vi "Event-Camera-amount.vi"(7 "# cameras":i32, 8 "error in (no error)":errorcluster, 10 "Data ref. in":refnum<data-value>, 11 "UI ref. in":refnum<data-value>) -> (0 "error out":errorcluster, 2 "Data ref.":refnum<data-value>, 3 "UI ref.":refnum<data-value>)   [LabVIEW 2013, in "CameraVision.lvlib" / "CV-UI.lvclass"]
uses:
  CV-UI.lvclass
  Main/CV-Main.lvclass
  Control-names.ctl
  Camera-selector.ctl
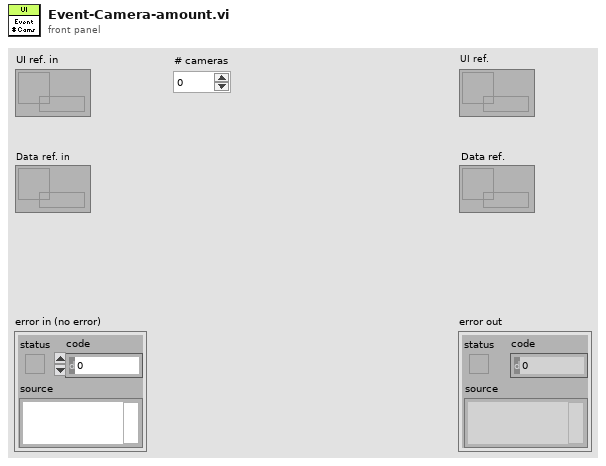
[diagram p1: front panel]
types:
  T1 = typedef "CameraVision.lvlib/CV-UI.lvclass/Control-names.ctl" = enum16{"Start acquisition", "Activate", "Stop acquisition", "Settings type", "Load settings", "Save settings", "Import images", "Camera selector", "Image type selector", "Batch browser", "Image refresh", "Parameter tabs", "Displays", "Processing tabs", "Processing selector", "Map characteristic", "Show info", "Manual trigger"}
  T2 = typedef "CameraVision.lvlib/CV-UI.lvclass/Camera-selector.ctl" = enum16{"Camera 1", "Camera 2"}
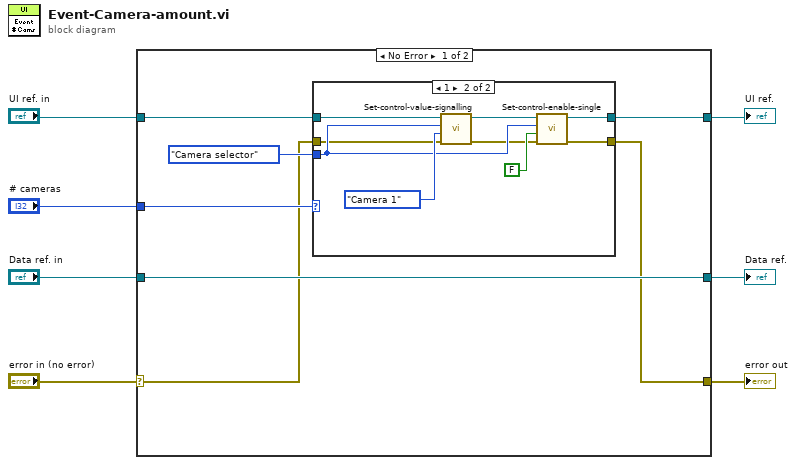
[diagram p0: block diagram]
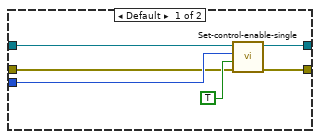
[diagram p2: hidden frame]
diagram:
  n1 = case shown="No Error" "error in (no error)" {
    selector: "error in (no error)" -> [w8 w32]
    tunnel: [w9 w32] -> w6
    tunnel: [w10 w31] -> w4
    tunnel: "UI ref. in" -> [w12 w31]
    tunnel: "Data ref. in" -> [w13 w30]
    tunnel: "# cameras" -> [w14 _]
    tunnel: [w13 w30] -> w2
    frame No Error {
      n2 = case shown="1" w14 {
        tunnel: w12 -> [w19 w29]
        tunnel: Control-names."Camera selector" ("Control name") -> [w17 w26]
        tunnel: [w18 w24] -> w10
        tunnel: [w16 w23] -> w9
        tunnel: w8 -> [w15 w21]
        frame Default {
          n3 = call "Set-control-enable-single.vi"("error in (no error)"=w15, "Enable?"=TRUE, "Control name"=w17, "UI ref. in"=w19) -> ("error out"=w16:errorcluster, "UI ref."=w18:refnum<data-value>)  [unwired: 6 in]
        }
        frame 1 {
          n4 = call "Set-control-value-signalling.vi"("error in (no error)"=w21, "Value"=Camera-selector."Camera 1" ("Camera"), "Control name"=w26, "UI ref. in"=w29) -> ("error out"=w22:errorcluster, "UI ref."=w28:refnum<data-value>)  [unwired: 6 in]
          n5 = call "Set-control-enable-single.vi"("error in (no error)"=w22, "Enable?"=FALSE, "Control name"=w26, "UI ref. in"=w28) -> ("error out"=w23:errorcluster, "UI ref."=w24:refnum<data-value>)  [unwired: 6 in]
        }
      }
    }
    frame Error {
    }
  }
  "error out" <- w6
  "Data ref." <- w2
  "UI ref." <- w4
